vi "Untitled 2.vi"() -> ()   [LabVIEW 2010]
uses:
  DLL-s/new_bsvt_test/Debug/new_bsvt_test.dll
panel:
  out "size(s)":i32
  out "arg1":cluster{"MSG":i16, "param":string, "Type":i16}[](array[cluster])
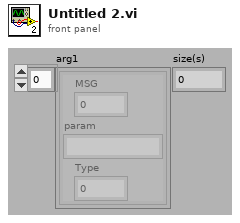
[diagram p1: front panel]
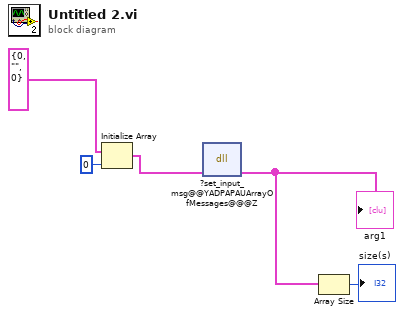
[diagram p0: block diagram]
diagram:
  n1 = Initialize Array(cluster{"MSG":i16, "param":string, "Type":i16} {"MSG"=0, "param"="", "Type"=0} ("Cluster"), 0 ("dimension size")) -> (w3:cluster{"MSG":i16, "param":string, "Type":i16}[])
  n2 = dll-call lib="D:/Liakh Tanya/Dissertation/Complex/DLL-s/new_bsvt_test/Debug/new_bsvt_test.dll" fn="?set_input_msg@@YADPAPAUArrayOfMessages@@@Z"("arg1"=w3) -> ("arg1"=w2:cluster{"MSG":i16, "param":string, "Type":i16}[])  [unwired: 4 in, 2 out]
  "arg1" <- w2
  n3 = Array Size(array=w2) -> (size(s)=→"size(s)":i32)
